vi "Analog Input - Synchronization.vi"() -> ()   [LabVIEW 2015]
doc: "This example demonstrates how to acquire a continuous amount of data (Waveform) using the DAQ device's internal clock. It also shows how to synchronize two devices for different device families (E Series, S Series, M Series, X Series, DSA, and SC Express), to simultaneously acquire the data.\n\nFor instructions on how to connect your signals to the DAQ device, refer to your device documentation."
uses:
  <vilib>/Utility/error.llb/DialogType.ctl
  <vilib>/DAQmx/write.llb/DAQmx Write (Analog 1D DBL 1Chan NSamp).vi
  <vilib>/DAQmx/read.llb/DAQmx Read (Analog 1D Wfm NChan NSamp).vi
  <vilib>/DAQmx/create/channels.llb/DAQmx Create Channel (AI-Voltage-Basic).vi
  <vilib>/DAQmx/configure/timing.llb/DAQmx Timing (Sample Clock).vi
  <vilib>/DAQmx/create/channels.llb/DAQmx Create Channel (AO-Voltage-Basic).vi
  <vilib>/DAQmx/configure/trigger.llb/DAQmx Start Trigger (Digital Edge).vi
  <vilib>/DAQmx/miscellaneous.llb/DAQmx Fill In Error Info.vi
  <resource>/objmgr/daqmx.rc
  <vilib>/Analysis/NI_AALBase.lvlib
panel:
  out "Numeric":i32=15
  in  "Slave Channels":tag="PXI1Slot2/ao0"
  in  "Synchronization Type*":T1(ring)=enum."DSA Reference Clock"
  in  "Stop":bool
  out "Waveform Graph":waveform(dbl)[](graph)=[{"t0"=timestamp(3635354447.0361495 s since 1904-01-01), "dt"=1.9999999995925458e-05, "Y"=array[25000 elements], "attributes"=variant("NI_ChannelName"=variant(string "PXI1Slot4/ai0"), "NI_UnitDescription"=variant(string "Volts"))}, {"t0"=timestamp(3635354447.0361495 s since 1904-01-01), "dt"=1.9999999995925458e-05, "Y"=array[25000 elements], "attributes"=variant("NI_ChannelName"=variant(string "PXI1Slot4/ai0"), "NI_UnitDescription"=variant(string "Volts"))}]
  in  "Sample Rate":dbl=50000.0
  in  "Master Physical Channel(s)":tag="PXI1Slot3/ai2"
  # "Channel Settings"
  # "Acquired Data"
  # "Timing Settings"
  # "*Note:  This example is intended to show low level synchronization of various devices.\nDSA, S Series, X Series, and SC Express devices support including channels from multiple devices in a single task.\nDAQmx automatically synchronizes the devices in such a task.  See the DAQmx Help>>\nDevice Considerations>>Multi Device Tasks section for further details."
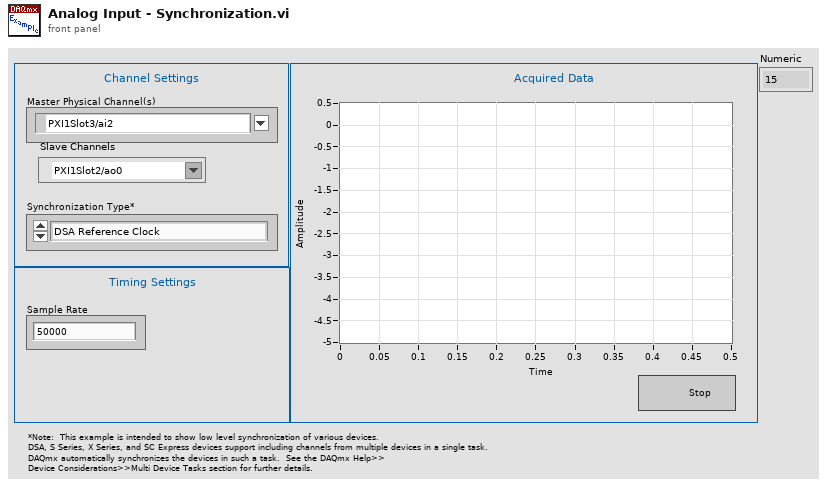
[diagram p1: front panel]
types:
  T1 = enum16{"E Series, S Series", "M Series (PCI)", "M Series (PXI)", "DSA Sample Clock Timebase", "DSA Reference Clock", "X Series (PCIe)", "X Series (PXIe), SC Express"}
  T2 = typedef "DialogType.ctl" = u16
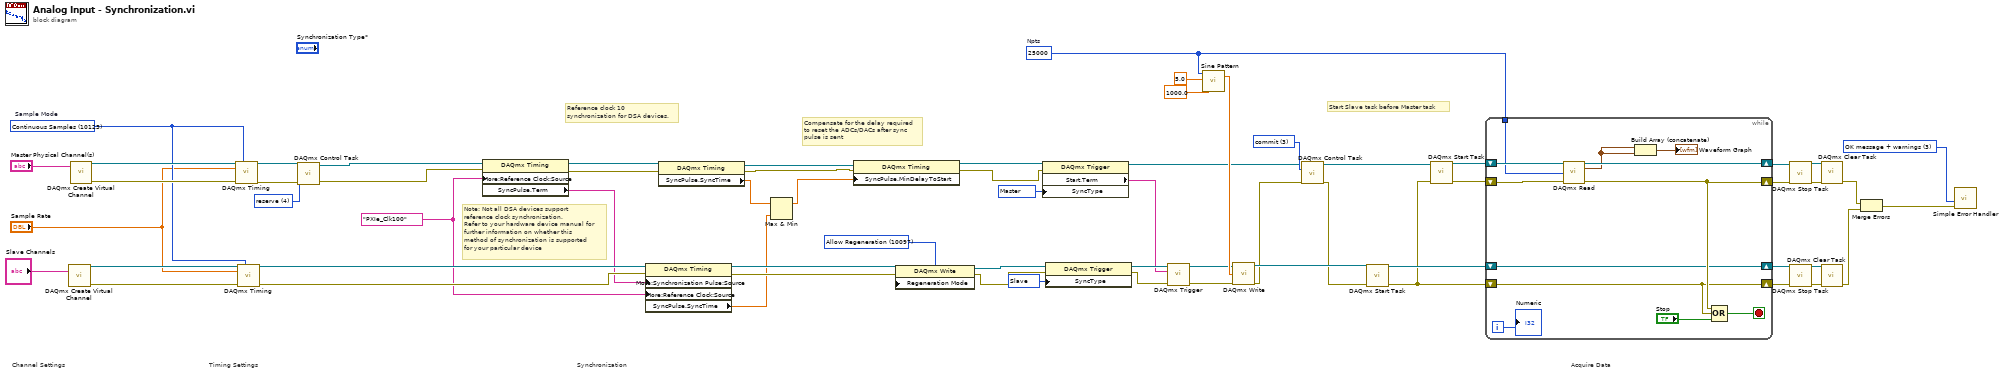
[diagram p0: block diagram]
diagram:
  w6 = 3 items=["verify"=2, "reserve"=4, "commit"=3, "unreserve"=5, "abort"=6] ("action")
  w17 = 10097 items=["Allow Regeneration"=10097, "Do Not Allow Regeneration"=10158] ("RegenMode")
  w20 = tag "PXIe_Clk100" ("RefClk.Src")
  w21 = 4 items=["verify"=2, "reserve"=4, "commit"=3, "unreserve"=5, "abort"=6] ("action")
  w26 = 15889 items=["None"=10230, "Master"=15888, "Slave"=15889] ("SyncType")
  w32 = 15888 items=["None"=10230, "Master"=15888, "Slave"=15889] ("SyncType")
  w35 = 25000  # Npts
  w40 = T2 3 items=["no dialog", "OK message", "continue or stop message", "OK message + warnings", "continue/stop + warnings"] ("type of dialog (OK msg:1)")
  w42 = 10123 items=["Finite Samples"=10178, "Continuous Samples"=10123, "Hardware Timed Single Point"=12522]  # Sample Mode
  # "Compensate for the delay required\nto reset the ADCs/DACs after sync\npulse is sent"
  # "Note: Not all DSA devices support\nreference clock synchronization.\nRefer to your hardware device manual for\nfurther information on whether this \nmethod of synchronization is supported\nfor your particular device"
  # "Reference clock 10\nsynchronization for DSA devices."
  # "Acquire Data"
  # "Synchronization"
  # "Timing Settings"
  # "Channel Settings"
  # "Start Slave task before Master task"
  n1 = call-poly <vilib>:"DAQmx Create Virtual Channel.vi"("physical channels"="Slave Channels") -> ("task out"=w44:refnum<k21>, "error out"=w46:errorcluster)  [unwired: 13 in]
  n2 = call-poly <vilib>:"DAQmx Create Virtual Channel.vi"("physical channels"="Master Physical Channel(s)") -> ("task out"=w48:refnum<k21>, "error out"=w47:errorcluster)  [unwired: 13 in]
  n3 = call-poly <vilib>:"DAQmx Timing.vi"("task/channels in"=w48, "sample mode"=w42, "rate"="Sample Rate", "error in"=w47) -> ("task out"=w25:refnum<k21>, "error out"=w22:errorcluster)  [unwired: 10 in]
  n4 = call-poly <vilib>:"DAQmx Timing.vi"("task/channels in"=w44, "sample mode"=w42, "rate"="Sample Rate", "error in"=w46) -> ("task out"=w45:refnum<k21>, "error out"=w43:errorcluster)  [unwired: 10 in]
  n5 = call <vilib>:"DAQmx Control Task.vi"("task/channels in"=w25, "action"=w21, "error in"=w22) -> ("task out"=w24:refnum<k21>, "error out"=w23:errorcluster)  [unwired: 11 in]
  n6 = property class="DAQmx Timing"(reference=w24, error in=w23, "More:Reference Clock:Source"=w20) -> (reference out=w15:refnum<k21>, error out=w12:errorcluster, "SyncPulse.Term"=w16:tag)
  n7 = property class="DAQmx Timing"(reference=w45, error in=w43, "More:Synchronization Pulse:Source"=w16, "More:Reference Clock:Source"=w20) -> (reference out=w19:refnum<k21>, error out=w18:errorcluster, "SyncPulse.SyncTime"=w10:dbl)
  n8 = property class="DAQmx Timing"(reference=w15, error in=w12) -> (reference out=w14:refnum<k21>, error out=w13:errorcluster, "SyncPulse.SyncTime"=w11:dbl)
  n9 = Max & Min(x=w11, y=w10) -> (max(x,y)=w9:dbl)  [unwired: 1 out]
  n10 = property class="DAQmx Timing"(reference=w14, error in=w13, "SyncPulse.MinDelayToStart"=w9) -> (reference out=w34:refnum<k21>, error out=w33:errorcluster)
  n11 = property class="DAQmx Write"(reference=w19, error in=w18, "Regeneration Mode"=w17) -> (reference out=w31:refnum<k21>, error out=w30:errorcluster)
  n12 = property class="DAQmx Trigger"(reference=w34, error in=w33, "SyncType"=w32) -> (reference out=w5:refnum<k21>, "Start.Term"=w27:tag)  [unwired: 1 out]
  n13 = property class="DAQmx Trigger"(reference=w31, error in=w30, "SyncType"=w26) -> (reference out=w29:refnum<k21>, error out=w28:errorcluster)
  n14 = call-poly <vilib>:"DAQmx Trigger.vi"("task/channels in"=w29, "source"=w27, "error in"=w28) -> ("task out"=w7:refnum<k21>, "error out"=w8:errorcluster)  [unwired: 11 in]
  n15 = call <vilib>:"Sine Pattern.vi"("cycles"=1000.0, "amplitude"=5.0, "samples"=w35) -> ("Sinusoidal Pattern"=w36:dbl[])  [unwired: 1 in, 1 out]
  n16 = call-poly <vilib>:"DAQmx Write.vi"("task/channels in"=w7, "data"=w36, "error in"=w8) -> ("task out"=w38:refnum<k21>, "error out"=w3:errorcluster)  [unwired: 10 in, 1 out]
  n17 = call <vilib>:"DAQmx Control Task.vi"("task/channels in"=w5, "action"=w6, "error in"=w3) -> ("task out"=w4:refnum<k21>, "error out"=w2:errorcluster)  [unwired: 11 in]
  n18 = call <vilib>:"DAQmx Start Task.vi"("task/channels in"=w38, "error in"=w2) -> ("task out"=w62:refnum<k21>, "error out"=w61:errorcluster)  [unwired: 12 in]
  n19 = call <vilib>:"DAQmx Start Task.vi"("task/channels in"=w4, "error in"=w61) -> ("task out"=w64:refnum<k21>, "error out"=w63:errorcluster)  [unwired: 12 in]
  n20 = while {
    shift-right: [w72] -> w59
    shift-left: w63 -> [w73]
    shift-right: [w68] -> w55
    shift-left: w61 -> [w68]
    shift-right: [w75] -> w60
    shift-left: w64 -> [w74]
    shift-right: [w69] -> w56
    shift-left: w62 -> [w69]
    tunnel: w35 -> [w66]
    i -> [w65]
    stop <- w76 stop-if-true
    n21 = call-poly <vilib>:"DAQmx Read.vi"("task/channels in"=w74, "number of samples per channel"=w66, "error in"=w73) -> ("task out"=w75:refnum<k21>, "data"=w67:waveform(dbl)[], "error out"=w72:errorcluster)  [unwired: 10 in]
    n22 = Build Array (concatenate)(w67, w67) -> (→"Waveform Graph":waveform(dbl)[])
    n23 = Compound Arithmetic op=OR(w72, w68, "Stop") -> (w76:bool)
    "Numeric" <- w65
  }
  n24 = call <vilib>:"DAQmx Stop Task.vi"("task/channels in"=w60, "error in"=w59) -> ("task out"=w57:refnum<k21>, "error out"=w58:errorcluster)  [unwired: 12 in]
  n25 = call <vilib>:"DAQmx Stop Task.vi"("task/channels in"=w56, "error in"=w55) -> ("task out"=w53:refnum<k21>, "error out"=w54:errorcluster)  [unwired: 12 in]
  n26 = call <vilib>:"DAQmx Clear Task.vi"("task in"=w57, "error in"=w58) -> ("error out"=w52:errorcluster)  [unwired: 13 in]
  n27 = call <vilib>:"DAQmx Clear Task.vi"("task in"=w53, "error in"=w54) -> ("error out"=w51:errorcluster)  [unwired: 13 in]
  n28 = Merge Errors(w52, w51) -> (w50:errorcluster)
  n29 = call <vilib>:"Simple Error Handler.vi"("type of dialog (OK msg:1)"=w40, "error in (no error)"=w50) -> ()  [unwired: 3 in, 5 out]
